vi "MOVING WINDOW Mean_Std DEV_SLOPE Ver01.vi"(5 "OLD Moving Window Values":dbl[](array[numeric]), 7 "OLD Time or Scan# Values\n(X-Values for SLOPE Calc)":dbl[](array[numeric]), 8 "error in":errorcluster, 10 "NEW Moving Window \nArray ELEMENT":dbl, 11 "NEW Moving Window \nTime Array ELEMENT":dbl) -> (0 "error out":errorcluster, 1 "MW SLOPE":dbl, 2 "MW Std. Dev.":dbl, 3 "MW Mean":dbl, 4 "NEW Moving Window Values":dbl[](array[numeric]), 6 "NEW Time or Scan# Values":dbl[](array[numeric]))   [LabVIEW 2017]
uses:
  <vilib>/Analysis/NI_AALBase.lvlib
  <vilib>/Analysis/NI_AALPro.lvlib
panel:
  out "XY Graph":cluster{"Y":dbl[], "Y":dbl[]}[](graph)
  # "Calculate the Mean and Standard Deviation of the Moving Window"
  # "New element is inserted into the fixed size array\nand the mean and std. dev. are calculated."
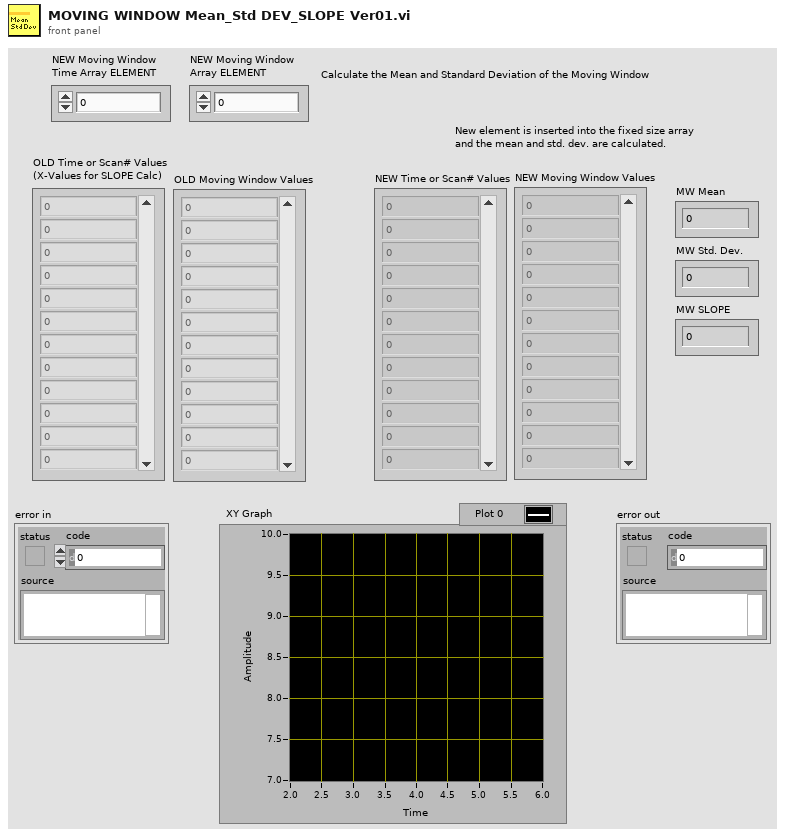
[diagram p1: front panel]
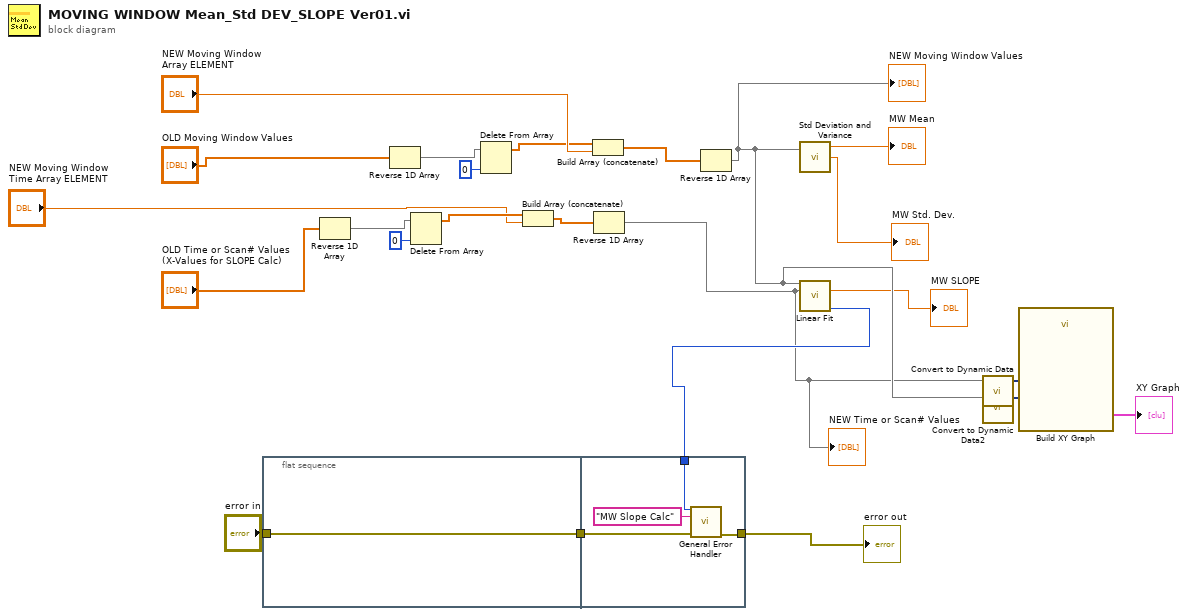
[diagram p0: block diagram]
diagram:
  n1 = flat-sequence {
    tunnel: "error in" -> [w25]
    tunnel: [w25] -> w14
    tunnel: [w27] -> w16
    tunnel: w14 -> [w28]
    tunnel: w13 -> [w26]
    frame #0 {
    }
    frame #1 {
      n2 = call <vilib>:"General Error Handler.vi"("[error code] (0)"=w26, "[error source] (\" \")"="MW Slope Calc" ("[error source] (\" \")"), "error in (no error)"=w28) -> ("error out"=w27:errorcluster)  [unwired: 8 in, 4 out]
    }
  }
  n3 = Reverse 1D Array(array="OLD Time or Scan# Values\n(X-Values for SLOPE Calc)") -> (reversed array=w7:dbl[])
  n4 = Reverse 1D Array(array="OLD Moving Window Values") -> (reversed array=w20:dbl[])
  n5 = Delete From Array(array=w7, index=0) -> (array with subset deleted=w5:dbl[])  [unwired: 1 in, 1 out]
  n6 = Delete From Array(array=w20, index=0) -> (array with subset deleted=w18:dbl[])  [unwired: 1 in, 1 out]
  n7 = Build Array (concatenate)(w5, "NEW Moving Window \nTime Array ELEMENT") -> (w2:dbl[])
  n8 = Build Array (concatenate)(w18, "NEW Moving Window \nArray ELEMENT") -> (w17:dbl[])
  n9 = Reverse 1D Array(array=w2) -> (reversed array=w1:dbl[])
  "NEW Time or Scan# Values" <- w1
  n10 = Reverse 1D Array(array=w17) -> (reversed array=w10:dbl[])
  "NEW Moving Window Values" <- w10
  n11 = call <vilib>:"Std Deviation and Variance.vi"("X"=w10) -> ("mean"=→"MW Mean":dbl, "standard deviation"=→"MW Std. Dev.":dbl)  [unwired: 1 in, 1 out]
  n12 = call <vilib>:"Linear Fit.vi"("Y"=w10, "X"=w1) -> ("slope"=→"MW SLOPE":dbl, "error"=w13:i32)  [unwired: 9 in, 3 out]
  n13 = call "Convert to Dynamic Data"("Array"=w1) -> ("Dynamic Data Type"=w11:dynamicdata)  [unwired: 3 in]
  n14 = call "Convert to Dynamic Data2"("Array"=w10) -> ("Dynamic Data Type"=w9:dynamicdata)  [unwired: 3 in]
  n15 = call "Build XY Graph"("Y Input"=w9, "X Input"=w11) -> ("XY Graph"=→"XY Graph":cluster{"X":dbl[], "Y":dbl[]}[])  [unwired: 8 in, 1 out]
  "error out" <- w16
